vi "V7310.Job.Set.vi"(6 "timeout ms (5000)":i32=5000, 8 "error in":errorcluster, 10 "Job":string, 11 "Connection in":refnum<k5>) -> (0 "error out":errorcluster, 3 "Connection out":refnum<k5>)   [LabVIEW 2016]
uses:
  LowLevel/V7310.Commands.ctl
panel:
  out "Data out":string
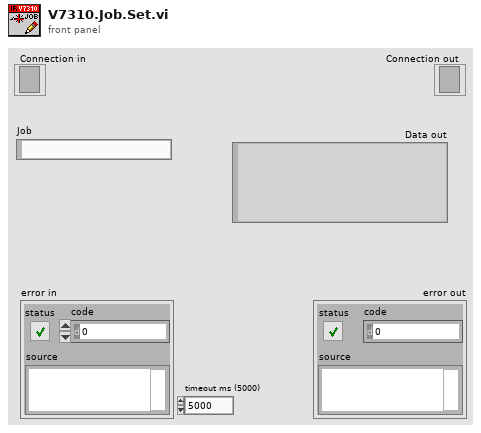
[diagram p1: front panel]
types:
  T1 = typedef "V7310.Commands.ctl" = enum16{"Start", "Stop", "GetStatus", "GetVarNames", "GetJobNames", "SetJob", "GetJob", "SetVars", "GetVars", "SetLayoutPosition", "SetRotation", "GetMessageID", "GetMessages", "ConfirmMessages", "DeleteMessages", "SetRTC", "GetRTC", "SetVarPosition", "SetIntensity", "GetIntensity", "SetStartTriggerDelay", "GetStartTriggerDelay", "SetStopTriggerDelay", "GetStopTriggerDelay", "SetConsecutiveTriggerDelay", "GetConsecutiveTriggerDelay", "SetMarkSpeed", "GetMarkSpeed"}
  T2 = typedef "V7310.ErrorLevels.ctl" = enum16{"OK", "Warning", "Error"}
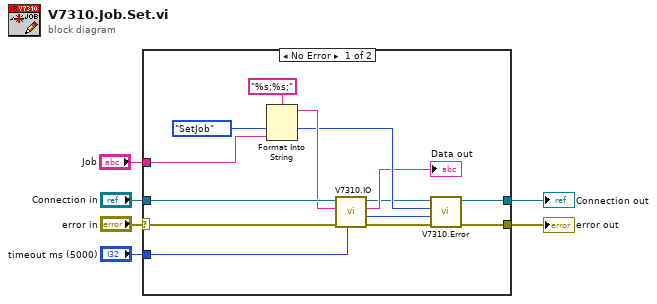
[diagram p0: block diagram]
diagram:
  n1 = case shown="No Error" "error in" {
    selector: "error in" -> [w17 w19]
    tunnel: "Connection in" -> [w18 w20]
    tunnel: [w7 w20] -> w5
    tunnel: "timeout ms (5000)" -> [w16 _]
    tunnel: [w8 w19] -> w2
    tunnel: "Job" -> [w10 _]
    frame No Error {
      w11 = V7310.Commands."SetJob" ("Cmd")
      n2 = Format Into String(format string="%s;%s;", w11, w10) -> (resulting string=w12:string)  [unwired: 2 in, 1 out]
      n3 = call "V7310.IO.vi"("timeout ms (5000)"=w16, "error in"=w17, "Data in"=w12, "Connection in"=w18) -> ("error out"=w14:errorcluster, "Error Level"=w15:T2, "Data out"=→"Data out":string, "Connection out"=w7:refnum<k5>)  [unwired: 4 in]
      n4 = call "V7310.Error.vi"("error in"=w14, "Error Level"=w15, "Cmd"=w11) -> ("error out"=w8:errorcluster)  [unwired: 8 in]
    }
    frame Error {
    }
  }
  "Connection out" <- w5
  "error out" <- w2
